vi "生成二维码.vi"(11 "条码数据":string="1234") -> (3 "图片":picture caption="新图片")   [LabVIEW 2012, in "条码.lvlib"]
uses:
  MakeQRBarcode.dll
panel:
  out "参数2":i32=4
  in  "图片名称":string="c:\\\\abc.bmp"
  in  "纠错等级":i32=2
  in  "掩模":i32
  in  "缩放参数":i32=4
  in  "条码版本":i32=3
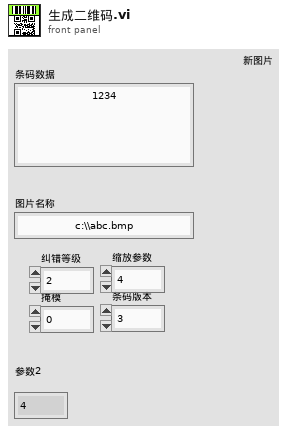
[diagram p1: front panel]
types:
  T1 = typedef "imagedata.ctl" = cluster{"image type":i32, "image depth":i32, "image":u8[], "mask":u8[], "colors":u32[], "Rectangle":cluster{"left":i16, "top":i16, "right":i16, "bottom":i16}}
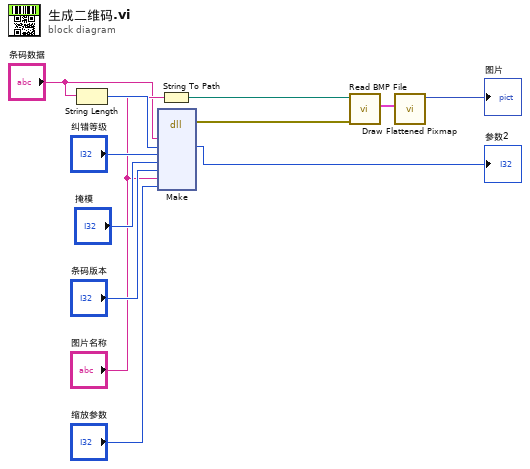
[diagram p0: block diagram]
diagram:
  n1 = String Length(string="条码数据") -> (length=w8:i32)
  n2 = dll-call lib="PTH1Habs FLABVIEWlabview使用库条码\t二维码MakeQRBarcode.dll" fn="Make"("条码数据"="条码数据", "条码数据长度"=w8, "纠错等级"="纠错等级", "掩模"="掩模", "条码样式"="条码版本", "图片文件名"="图片名称", "缩放"="缩放参数") -> (error out=w4:errorcluster, "条码数据长度"=→"参数2":i32)  [unwired: 10 in, 1 out]
  n3 = String To Path(string="图片名称") -> (path=w3:path)
  n4 = call <vilib>:"Read BMP File.vi"("error in (no error)"=w4, "path to BMP file"=w3) -> ("image data"=w2:T1)  [unwired: 7 in, 2 out]
  n5 = call <vilib>:"Draw Flattened Pixmap.vi"("image data"=w2) -> ("new picture"=→"图片":picture)  [unwired: 8 in]
